vi "190627_PDFF.vi"() -> ()   [LabVIEW 2019]
uses:
  <vilib>/rvi/interface/nirviReadWriteControl/nirviReadWriteControl.xnode
  <vilib>/rvi/interface/Simulation/niFpgaSimulationCallBeginRW.vi
  <vilib>/rvi/errors/niLvFpgaAdjustHostInterfaceError.vi
  <vilib>/rvi/interface/nirviMethod/nirviMethod.xnode
  <vilib>/FPGAPlugInAG/Dynamic/niLvFpga_Reset_Dynamic.vi
  <vilib>/FPGAPlugInAG/Dynamic/niLvFpga_Run_Dynamic.vi
  <vilib>/rvi/interface/nirviCloseFPGA/nirviCloseFPGA.xnode
  <vilib>/Platform/TimedLoop/XDataNode/XDataNode.xnode
  <vilib>/Platform/TimedLoop/XDataNode/nitl_modes.ctl
  <vilib>/Platform/TimedLoop/XDataNode/XDNodeRunTimeDep.lvlib
  <vilib>/Platform/TimedLoop/XDataNode/wakeup.ctl
  <vilib>/Platform/TimedLoop/XDataNode/timing_clust.ctl
  <vilib>/rvi/interface/nirviOpenFPGA/nirviOpenFPGA.xnode
  <vilib>/Utility/Variable/NI_VariableUtilities.lvlib
  FPGA_TwoAxisEncoder_revised.vi
  <vilib>/FPGAPlugInAG/Dynamic/niLvFpga_Close_Dynamic.vi
panel:
  out "Time Slots (sec)":dbl[](array[numeric])
  out "All times (sec)":dbl
  out "one period  length":i32
  out "one period start time":i32
  in  "HOST Sample Rate (Hz)":i32=1000
  in  "LOAD":bool
  out "(LS) RMS X (one) (um)":dbl format="%0.4f"
  out "(LS) MAX ERROR X (um)":dbl format="%0.4f"
  out "(LS) RMS ERROR X (um)":dbl format="%0.4f"
  out "(En) RMS X (one) (um)":dbl format="%0.4f"
  out "(LS) RMS Z (one) (um)":dbl format="%0.4f"
  out "(LS) MAX ERROR Z (um)":dbl format="%0.4f"
  out "(LS) RMS ERROR Z (um)":dbl format="%0.4f"
  out "CMD X (rpm)":dbl[](graph)
  out "Linear Scale Position X (mm)":dbl[](graph)
  out "Linear Scale Position Z (mm)":dbl[](graph)
  out "(En) RMS Z (one) (um)":dbl format="%0.4f"
  out "CMD Z (rpm)":dbl[](graph)
  out "Position X (mm)":dbl[](graph)
  out "Linear Scale Position Error X (um)":dbl[](graph)
  out "Linear Scale Position Error Z (um)":dbl[](graph)
  out "Delay":i32
  out "(En) MAX ERROR X (um)":dbl format="%0.4f"
  out "(En) RMS ERROR X (um)":dbl format="%0.4f"
  out "Encoder Position Error X (um)":dbl[](graph)
  out "Position Command X (mm)":dbl[](graph)
  out "(En) MAX ERROR Z (um)":dbl format="%0.4f"
  out "(En) RMS ERROR Z (um)":dbl format="%0.4f"
  out "Encoder Position Error Z (um)":dbl[](graph)
  in  "RUN":bool
  in  "CLEAR":bool
  out "V Loop":bool
  out "Length(Response)":i32
  out "Length(Command)":i32
  out "Done":bool
  out "Error Out (FPGA)":errorcluster
  out "Error Out (Host)":errorcluster
  out "Position Z (mm)":dbl[](graph)
  out "FPGA INITIALIZED":bool
  in  "FPGA Sample Rate (Hz)":dbl=100000.0
  out "Position Command Z (mm)":dbl[](graph)
  in  "STOP":bool
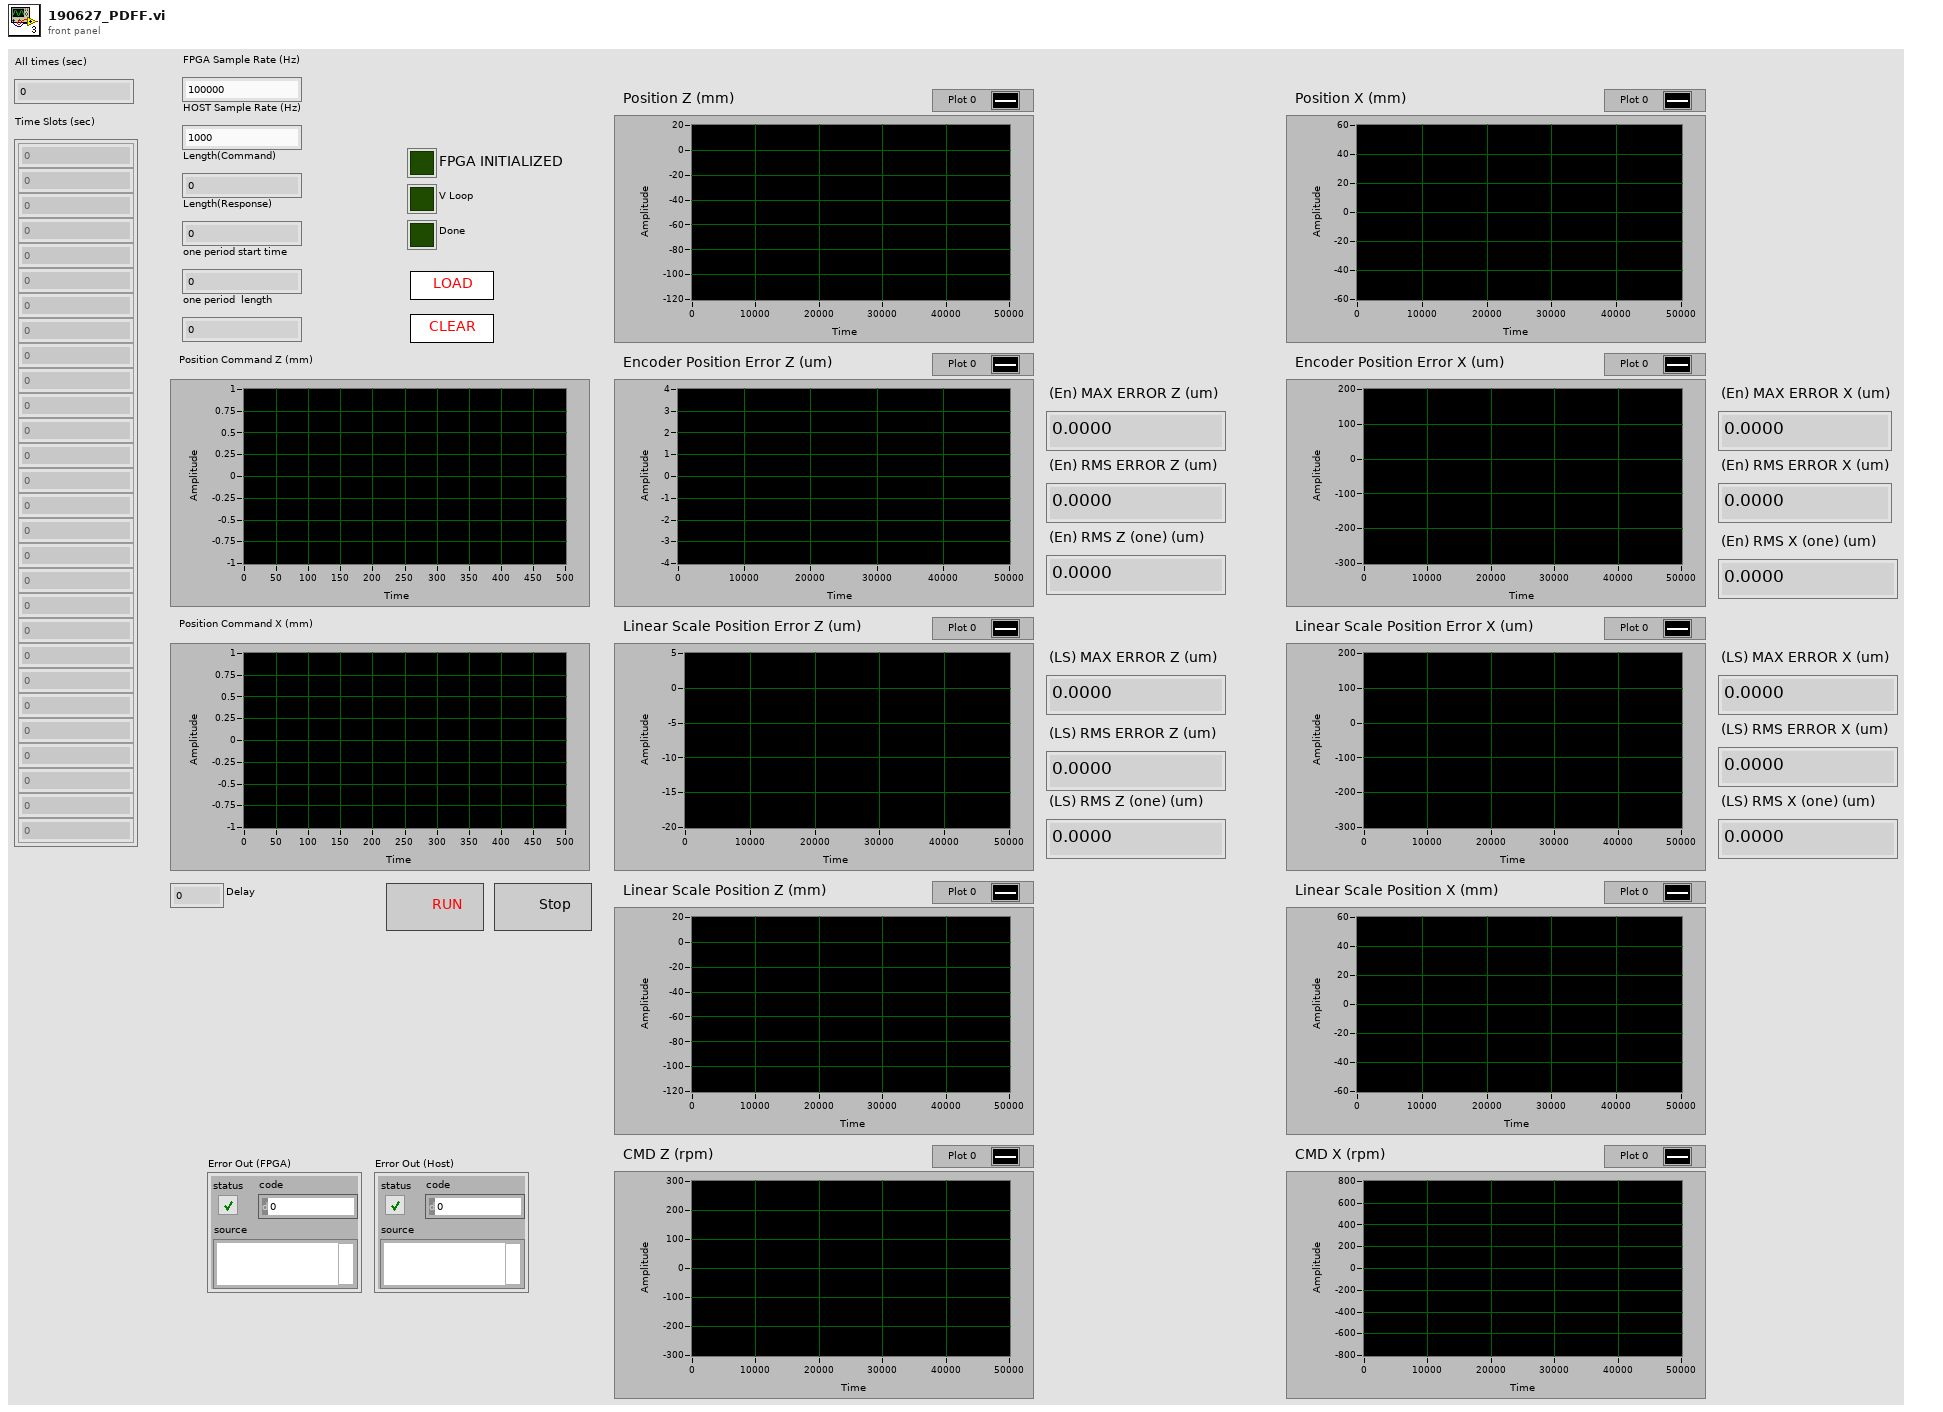
[diagram p1: front panel]
types:
  T1 = typedef "XDNodeRunTimeDep.lvlib/timing_clust.ctl" = cluster{"Expected End [f-1]":u64, "Actual End [f-1]":u64, "Finished Late? [f-1]":bool, "Expected End [i-1]":u64, "Actual End [i-1]":u64, "Finished Late? [i-1]":bool, "Expected Start [i]":u64, "Actual Start [i]":u64, "Expected Start [f]":u64, "Actual Start [f]":u64, "Source Name":string, "Structure Name":string, "Period":i64, "Deadline":i64, "Offset":i64, "Start":i64, "Priority":i32, "Timeout":i32, "Mode":T2, "Wakeup Reason":T3, "Error":errorcluster, "Source Type":string, "Secondary Source Type":string, "Global End Time":u64, "Global Start Time":u64, "Frame Duration":u64, "Iteration Duration":u64, "Assigned CPU":i32, "I/O Scan Engine Mode":u32}
  T2 = typedef "XDNodeRunTimeDep.lvlib/nitl_modes.ctl" = enum32{"No Change", "Process missed periods, maintain original phase", "Discard missed periods, maintain original phase", "Process missed periods, ignore original phase", "Discard missed periods, ignore original phase"}
  T3 = typedef "XDNodeRunTimeDep.lvlib/wakeup.ctl" = enum32{"Normal", "Aborted", "Asynchronous wakeup", "Timing source error", "Timed loop error", "Timeout"}
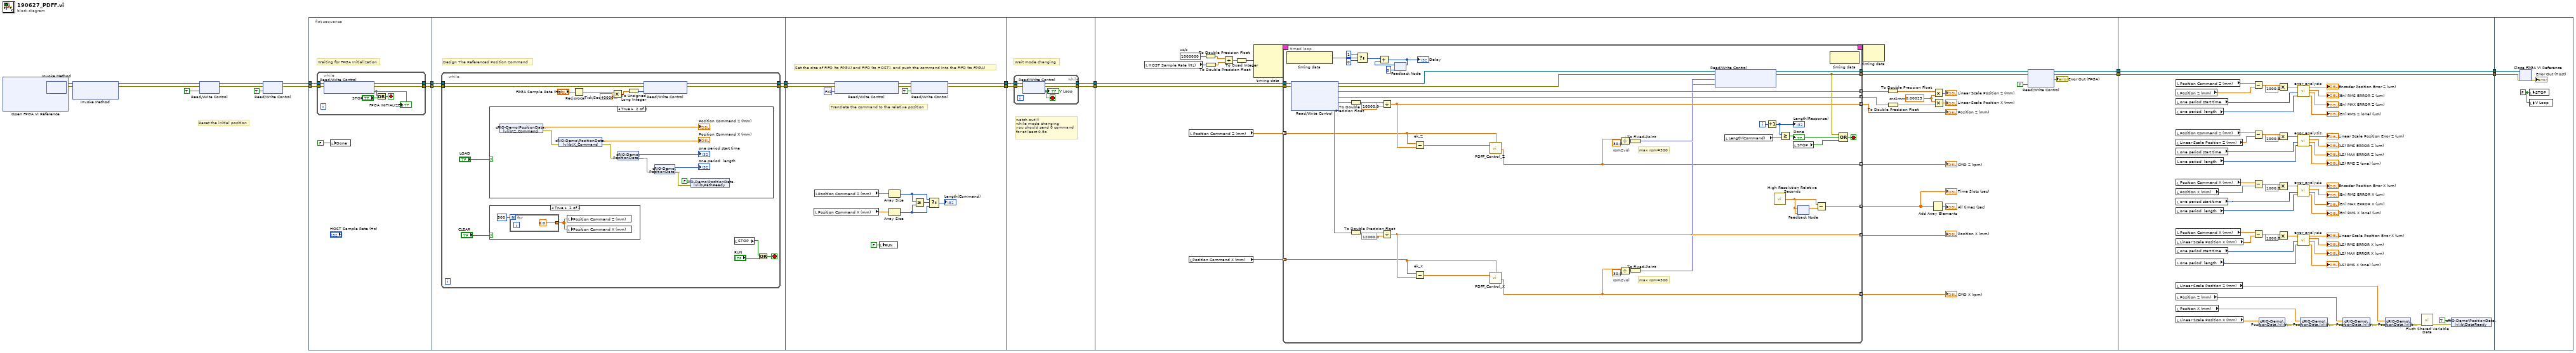
[diagram p0: block diagram]
diagram:
  # "Reset the initial position"
  n1 = xnode "Open FPGA VI Reference"() -> ("FPGA VI Reference Out"=w7:refnum<k20>, "error out"=w6:errorcluster)  [unwired: 2 in]
  n2 = xnode "Invoke Method"("FPGA VI Reference In"=w7, "error in"=w6) -> ("FPGA VI Reference Out"=w20:refnum<k20>, "error out"=w19:errorcluster)
  n3 = xnode "Invoke Method"("FPGA VI Reference In"=w20, "error in"=w19) -> ("FPGA VI Reference Out"=w5:refnum<k20>, "error out"=w4:errorcluster)  [unwired: 1 in]
  n4 = xnode "Read/Write Control"("FPGA VI Reference In"=w5, "error in"=w4, "Initial"=TRUE ("Reset Encoder")) -> ("FPGA VI Reference Out"=w3:refnum<k20>, "error out"=w2:errorcluster)
  n5 = xnode "Read/Write Control"("FPGA VI Reference In"=w3, "error in"=w2, "Start"=TRUE) -> ("FPGA VI Reference Out"=w14:refnum<k20>, "error out"=w13:errorcluster)
  n6 = flat-sequence {
    tunnel: w14 -> [w29]
    tunnel: w13 -> [w28]
    tunnel: [w27] -> w24
    tunnel: [w26] -> w23
    tunnel: w24 -> [w40]
    tunnel: w23 -> [w39]
    tunnel: [w38] -> w22
    tunnel: [w37] -> w21
    tunnel: w22 -> [w76]
    tunnel: [w79] -> w18
    tunnel: w21 -> [w75]
    tunnel: [w78] -> w16
    tunnel: w18 -> [w83]
    tunnel: [w81] -> w17
    tunnel: w16 -> [w82]
    tunnel: [w80] -> w15
    tunnel: w17 -> [w119]
    tunnel: [w116] -> w11
    tunnel: w15 -> [w118]
    tunnel: [w109] -> w8
    tunnel: w11 -> [w226]
    tunnel: [w226] -> w10
    tunnel: [w225] -> w9
    tunnel: w8 -> [w225]
    tunnel: w10 -> [w229]
    tunnel: w9 -> [w228]
    frame #0 {
      # "Waiting for FPGA Initialization"
      n7 = while {
        tunnel: w29 -> [w36]
        tunnel: w28 -> [w33]
        tunnel: [w32] -> w26
        tunnel: [w31] -> w27
        stop <- w35 stop-if-true
        n8 = xnode "Read/Write Control"("FPGA VI Reference In"=w36, "error in"=w33) -> ("FPGA VI Reference Out"=w31:refnum<k20>, "error out"=w32:errorcluster, "SYSTEM INITIALIZED"=w30)
        "FPGA INITIALIZED" <- w30
        n9 = Or(x=w30, y="STOP") -> (x .or. y?=w35:bool)
      }
      n10 = local write "Done"(FALSE ("Done")) -> ()
    }
    frame #1 {
      # "Design The Referenced Position Command"
      n11 = while {
        tunnel: w40 -> [w54]
        tunnel: w39 -> [w53]
        tunnel: [w48] -> w38
        tunnel: [w47] -> w37
        stop <- w46 stop-if-true
        w50 = 40000000.0  # Tick/Sec
        n12 = case shown="True" "LOAD" {
          frame False {
          }
          frame True {
            n13 = shared-variable "cRIO-Demo\\PositionData.lvlib\\Z_Command"() -> (→"Position Command Z (mm)":dbl[], error out=w65:errorcluster)  [unwired: 1 in]
            n14 = shared-variable "cRIO-Demo\\PositionData.lvlib\\X_Command"(error in=w65) -> (→"Position Command X (mm)":dbl[], error out=w61:errorcluster)
            n15 = shared-variable "cRIO-Demo\\PositionData.lvlib\\t0"(error in=w61) -> (→"one period start time":i32, error out=w62:errorcluster)
            n16 = shared-variable "cRIO-Demo\\PositionData.lvlib\\tL"(error in=w62) -> (→"one period  length":i32, error out=w60:errorcluster)
            n17 = shared-variable "cRIO-Demo\\PositionData.lvlib\\PathReady"(FALSE ("PathReady"), error in=w60) -> ()  [unwired: 1 out]
          }
        }
        n18 = case shown="True" "CLEAR" {
          frame False {
          }
          frame True {
            n19 = for {
              N: 500 -> [_]
              tunnel: [0.0 ("element")] -> w56 mode=indexing
            }
            n20 = local write "Position Command Z (mm)"(w56) -> ()
            n21 = local write "Position Command X (mm)"(w56) -> ()
          }
        }
        n22 = Reciprocal(x="FPGA Sample Rate (Hz)") -> (1/x=w51:dbl)
        n23 = Multiply(x=w51, y=w50) -> (x*y=w52:dbl)
        n24 = To Unsigned Long Integer(number=w52) -> (unsigned 32bit integer=w49:u32)
        n25 = xnode "Read/Write Control"("FPGA VI Reference In"=w54, "error in"=w53, "Loop Delay (Tick)"=w49) -> ("FPGA VI Reference Out"=w48:refnum<k20>, "error out"=w47:errorcluster)
        n26 = local read "STOP"() -> (w45:bool)
        n27 = Or(x=w45, y="RUN") -> (x .or. y?=w46:bool)
      }
    }
    frame #2 {
      # "Translate the command to the relative position"
      # "Set the size of FIFO (to FPGA) and FIFO (to HOST), and push the command into the FIFO (to FPGA)"
      n28 = local read "Position Command X (mm)"() -> (w67:dbl[])
      n29 = local read "Position Command Z (mm)"() -> (w68:dbl[])
      n30 = xnode "Read/Write Control"("FPGA VI Reference In"=w76, "Output Votage Bound (vol)"=fxp<+,20,5> 10.0) -> ()  [unwired: 1 in, 2 out]
      n31 = local write "RUN"(FALSE) -> ()
      n32 = Array Size(array=w68) -> (size(s)=w71:i32)
      n33 = Array Size(array=w67) -> (size(s)=w70:i32)
      n34 = xnode "Read/Write Control"("FPGA VI Reference In"=w76, "error in"=w75, "HOST READY?"=TRUE) -> ("FPGA VI Reference Out"=w79:refnum<k20>, "error out"=w78:errorcluster)
      n35 = Greater Or Equal?(x=w71, y=w70) -> (x >= y?=w72:bool)
      n36 = Select(t=w71, s=w72, f=w70) -> (s? t:f=→"Length(Command)":i32)
    }
    frame #3 {
      # "watch out!!!\nwhile mode changing\nyou should send 0 command\nfor at least 0.5s."
      # "Wait mode changing"
      n37 = while {
        tunnel: w83 -> [w88]
        tunnel: w82 -> [w87]
        tunnel: [w86] -> w81
        tunnel: [w85] -> w80
        stop <- w84 stop-if-true
        n38 = xnode "Read/Write Control"("FPGA VI Reference In"=w88, "error in"=w87) -> ("FPGA VI Reference Out"=w86:refnum<k20>, "error out"=w85:errorcluster, "V Loop"=w84)
        "V Loop" <- w84
      }
    }
    frame #4 {
      w91 = 0.00025  # cnt2mm
      w113 = 1000000  # us/s
      n39 = local read "HOST Sample Rate (Hz)"() -> (w102:i32)
      n40 = local read "Position Command X (mm)"() -> (w100:dbl[])
      n41 = local read "Position Command Z (mm)"() -> (w101:dbl[])
      n42 = To Double Precision Float(number=w113) -> (double precision float=w105:dbl)
      n43 = To Double Precision Float(number=w102) -> (double precision float=w106:dbl)
      n44 = Divide(x=w105, y=w106) -> (x/y=w112:dbl)
      n45 = To Quad Integer(1:w112) -> (0:w111:i64)
      n46 = node-c288(w111) -> (w115:T1)  [unwired: 3 in]
      n47 = timed-loop {
        tunnel: w119 -> [w147]
        tunnel: w118 -> [w145]
        tunnel: [w131] -> w117
        timing: w115 -> [_]
        timing-out: [_] -> w114
        tunnel: [w130] -> w110
        tunnel: [w141] -> w96 mode=indexing
        tunnel: [w138] -> w94 mode=indexing
        tunnel: [w123] -> w103 mode=indexing
        tunnel: [w142] -> w95 mode=indexing
        tunnel: w101 -> [w124] mode=indexing
        tunnel: w100 -> [w121] mode=indexing
        tunnel: [w120] -> w99 mode=indexing
        tunnel: [w136] -> w93 mode=indexing
        tunnel: [w126] -> w89 mode=indexing
        i -> [w158]
        stop <- w163 stop-if-true
        w140 = 30.0  # rpm2vol
        w159 = 30.0  # rpm2vol
        # "max rpm=300"
        # "max rpm=300"
        n48 = node-c288() -> (w152:bool)  [unwired: 1 in]
        n49 = xnode "Read/Write Control"("FPGA VI Reference In"=w147, "error in"=w145) -> ("FPGA VI Reference Out"=w135:refnum<k20>, "error out"=w134:errorcluster, "Line Scale Z (count)"=w138, "Line Scale X (count)"=w136, "Encoder Z (count)"=w137, "Encoder X (count)"=w129)
        n50 = To Double Precision Float(number=w137) -> (double precision float=w157:dbl)
        n51 = To Double Precision Float(number=w129) -> (double precision float=w144:dbl)
        n52 = Select(t=1, s=w152, f=0) -> (s? t:f=w151:i32)
        n53 = Divide(x=w157, y=10000.0) -> (x/y=w141:dbl)
        n54 = Divide(x=w144, y=12000.0) -> (x/y=w142:dbl)
        n55 = feedback #1(0) -> (w149:i32)
        n56 = Add(x=w151, y=w149) -> (x+y=w150:i32)
        "Delay" <- w150
        n57 = feedback-in #1(w150) -> ()
        n58 = Subtract "ek_Z"(x=w124, y=w141) -> (x-y=w125:dbl)
        n59 = Subtract "ek_X"(x=w121, y=w142) -> (x-y=w122:dbl)
        n60 = call "PDFF_Control_Z.vi"("e(k)"=w125, "r(k)"=w124) -> ("u(k)"=w123:dbl)  [unwired: 4 in, 1 out]
        n61 = call "PDFF_Control_X.vi"("e(k)"=w122, "r(k)"=w121) -> ("u(k)"=w120:dbl)  [unwired: 4 in, 1 out]
        n62 = Divide(x=w123, y=w159) -> (x/y=w160:fxp<+/-,20,5>)
        n63 = Divide(x=w120, y=w140) -> (x/y=w139:fxp<+/-,20,5>)
        n64 = To Fixed-Point(number=w160) -> (fixed-point=w133:fxp<+/-,20,5>)  [unwired: 1 in]
        n65 = To Fixed-Point(number=w139) -> (fixed-point=w132:fxp<+/-,20,5>)  [unwired: 1 in]
        n66 = xnode "Read/Write Control"("FPGA VI Reference In"=w135, "error in"=w134, "Velocity Command Z (vol)"=w133, "Velocity Command X (vol)"=w132) -> ("FPGA VI Reference Out"=w131:refnum<k20>, "error out"=w130:errorcluster)
        n67 = local read "Length(Command)"() -> (w146:i32)
        n68 = Increment(x=w158) -> (x+1=w155:i32)
        "Length(Response)" <- w155
        n69 = call <vilib>:"High Resolution Relative Seconds.vi"() -> ("relative seconds"=w128:dbl)
        n70 = Greater Or Equal?(x=w155, y=w146) -> (x >= y?=w162:bool)
        "Done" <- w162
        n71 = local read "STOP"() -> (w161:bool)
        n72 = feedback #2(w128) -> (w127:dbl)
        n73 = feedback-in #2(w128) -> ()
        n74 = Subtract(x=w128, y=w127) -> (x-y=w126:dbl)
        n75 = node-c288() -> ()  [unwired: 1 in, 1 out]
        n76 = Compound Arithmetic op=OR(w130, w162, w161) -> (w163:bool)
      }
      "Position Z (mm)" <- w96
      "Position X (mm)" <- w95
      "CMD Z (rpm)" <- w103
      "CMD X (rpm)" <- w99
      "Time Slots (sec)" <- w89
      n77 = node-c288(w114) -> ()  [unwired: 1 out]
      n78 = To Double Precision Float(number=w94) -> (double precision float=w92:dbl[])
      n79 = To Double Precision Float(number=w93) -> (double precision float=w98:dbl[])
      n80 = Add Array Elements(numeric array=w89) -> (sum=→"All times (sec)":dbl)
      n81 = Multiply(x=w92, y=w91) -> (x*y=→"Linear Scale Position Z (mm)":dbl[])
      n82 = Multiply(x=w91, y=w98) -> (x*y=→"Linear Scale Position X (mm)":dbl[])
      n83 = xnode "Read/Write Control"("FPGA VI Reference In"=w117, "error in"=w110, "stop"=TRUE) -> ("FPGA VI Reference Out"=w116:refnum<k20>, "error out"=w109:errorcluster, "Error Out"=→"Error Out (FPGA)")
    }
    frame #5 {
      n84 = local read "Position Command Z (mm)"() -> (w224:dbl[])
      n85 = local read "Position Z (mm)"() -> (w223:dbl[])
      n86 = local read "one period start time"() -> (w214:i32)
      n87 = local read "one period  length"() -> (w213:i32)
      n88 = local read "Position Command Z (mm)"() -> (w177:dbl[])
      n89 = local read "Linear Scale Position Z (mm)"() -> (w220:dbl[])
      n90 = local read "one period start time"() -> (w208:i32)
      n91 = local read "one period  length"() -> (w207:i32)
      n92 = local read "Position Command X (mm)"() -> (w195:dbl[])
      n93 = local read "Position X (mm)"() -> (w194:dbl[])
      n94 = local read "one period start time"() -> (w193:i32)
      n95 = local read "one period  length"() -> (w192:i32)
      n96 = local read "Position Command X (mm)"() -> (w178:dbl[])
      n97 = local read "Linear Scale Position X (mm)"() -> (w191:dbl[])
      n98 = local read "one period start time"() -> (w190:i32)
      n99 = local read "one period  length"() -> (w189:i32)
      n100 = local read "Linear Scale Position Z (mm)"() -> (w187:dbl[])
      n101 = local read "Position Z (mm)"() -> (w179:dbl[])
      n102 = local read "Position X (mm)"() -> (w180:dbl[])
      n103 = local read "Linear Scale Position X (mm)"() -> (w188:dbl[])
      n104 = Subtract(x=w224, y=w223) -> (x-y=w221:dbl[])
      n105 = Subtract(x=w177, y=w220) -> (x-y=w172:dbl[])
      n106 = Subtract(x=w195, y=w194) -> (x-y=w205:dbl[])
      n107 = Subtract(x=w178, y=w191) -> (x-y=w176:dbl[])
      n108 = shared-variable "cRIO-Demo\\PositionData.lvlib\\X_LS"(w188) -> (error out=w186:errorcluster)  [unwired: 1 in]
      n109 = Multiply(x=w221, y=1000.0) -> (x*y=w219:dbl[])
      n110 = Multiply(x=w172, y=1000.0) -> (x*y=w171:dbl[])
      n111 = Multiply(x=w205, y=1000.0) -> (x*y=w206:dbl[])
      n112 = Multiply(x=w176, y=1000.0) -> (x*y=w174:dbl[])
      n113 = call "error_analysis.vi"("tLength"=w213, "t0"=w214, "data in (um)"=w219) -> ("rms (one) (um)"=→"(En) RMS Z (one) (um)":dbl, "max err (um)"=→"(En) MAX ERROR Z (um)":dbl, "rms (all) (um)"=→"(En) RMS ERROR Z (um)":dbl, "data out (um)"=→"Encoder Position Error Z (um)":dbl[])  [unwired: 5 in]
      n114 = call "error_analysis.vi"("tLength"=w207, "t0"=w208, "data in (um)"=w171) -> ("rms (one) (um)"=→"(LS) RMS Z (one) (um)":dbl, "max err (um)"=→"(LS) MAX ERROR Z (um)":dbl, "rms (all) (um)"=→"(LS) RMS ERROR Z (um)":dbl, "data out (um)"=→"Linear Scale Position Error Z (um)":dbl[])  [unwired: 5 in]
      n115 = call "error_analysis.vi"("tLength"=w192, "t0"=w193, "data in (um)"=w206) -> ("rms (one) (um)"=→"(En) RMS X (one) (um)":dbl, "max err (um)"=→"(En) MAX ERROR X (um)":dbl, "rms (all) (um)"=→"(En) RMS ERROR X (um)":dbl, "data out (um)"=→"Encoder Position Error X (um)":dbl[])  [unwired: 5 in]
      n116 = call "error_analysis.vi"("tLength"=w189, "t0"=w190, "data in (um)"=w174) -> ("rms (one) (um)"=→"(LS) RMS X (one) (um)":dbl, "max err (um)"=→"(LS) MAX ERROR X (um)":dbl, "rms (all) (um)"=→"(LS) RMS ERROR X (um)":dbl, "data out (um)"=→"Linear Scale Position Error X (um)":dbl[])  [unwired: 5 in]
      n117 = shared-variable "cRIO-Demo\\PositionData.lvlib\\X_EN"(w180, error in=w186) -> (error out=w185:errorcluster)
      n118 = shared-variable "cRIO-Demo\\PositionData.lvlib\\Z_EN"(w179, error in=w185) -> (error out=w184:errorcluster)
      n119 = shared-variable "cRIO-Demo\\PositionData.lvlib\\Z_LS"(w187, error in=w184) -> (error out=w183:errorcluster)
      n120 = call <vilib>:"Flush Shared Variable Data.vi"("error in (no error)"=w183) -> ("error out"=w182:errorcluster)  [unwired: 10 in]
      n121 = shared-variable "cRIO-Demo\\PositionData.lvlib\\DataReady"(TRUE, error in=w182) -> ()  [unwired: 1 out]
    }
    frame #6 {
      w227 = FALSE ("STOP")
      n122 = xnode "Close FPGA VI Reference"("FPGA VI Reference In"=w229, "error in"=w228) -> ("error out"=→"Error Out (Host)":errorcluster)
      n123 = local write "STOP"(w227) -> ()
      n124 = local write "V Loop"(w227) -> ()
    }
  }
